vi "新写入PN.vi"(0 "产品名":string, 1 "测温功能":string, 2 "预留（默认XX）":string="XX", 5 "分辨率":string, 7 "镜头":string, 9 "增益模式":string, 11 "error in":errorcluster, 12 "产品料号":string) -> (4 "return":i32, 15 "error out":errorcluster)   [LabVIEW 2016]
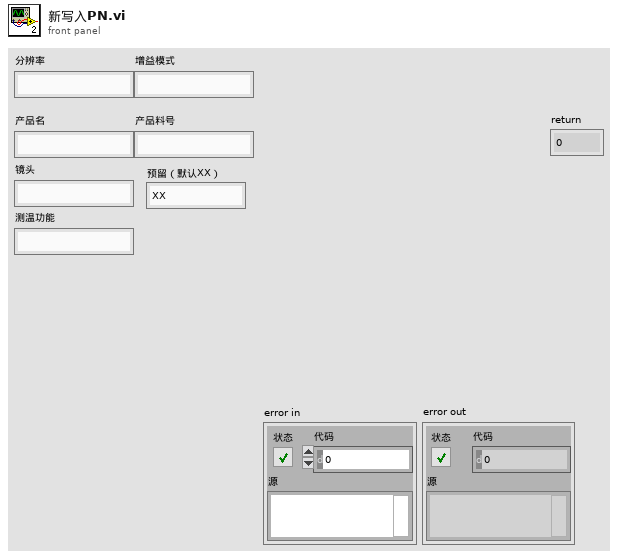
[diagram p1: front panel]
types:
  T1 = cluster{"byCmdType":u8, "bySubCmd":u8, "byPara":u8, "byAddr_h":u8, "byAddr_l":u8, "byAddr_ll":u8, "byLen_h":u8, "byLen_l":u8}
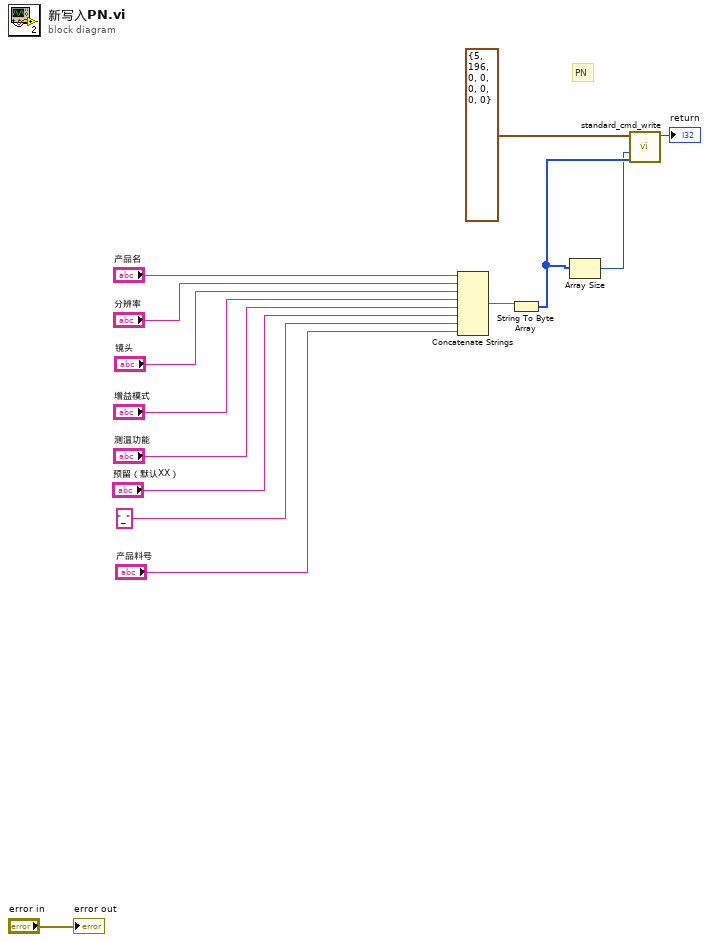
[diagram p0: block diagram]
diagram:
  # "PN"
  n1 = Concatenate Strings("产品名", "分辨率", "镜头", "增益模式", "测温功能", "预留（默认XX）", "_" ("string"), "产品料号") -> (w10:string)
  n2 = String To Byte Array(string=w10) -> (unsigned byte array=w9:u8[])
  n3 = Array Size(array=w9) -> (size(s)=w8:i32)
  n4 = call "standard_cmd_write.vi"("data"=w9, "dwLen"=w8, "cmd_std_header_t"=T1 {"byCmdType"=5, "bySubCmd"=196, "byPara"=0, "byAddr_h"=0, "byAddr_l"=0, "byAddr_ll"=0, "byLen_h"=0, "byLen_l"=0}) -> ("return"=→"return":i32)  [unwired: 7 in, 1 out]
  "error out" <- "error in"
